vi "test purge with argon.vi"() -> ()   [LabVIEW 2017]
uses:
  <instrlib>/Harvard Apparatus PHD Ultra Series/Harvard Apparatus PHD Ultra Series.lvlib
panel:
  in  "VISA resource name":refnum<visa-resource-name>="COM12"
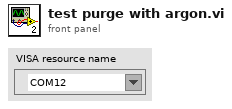
[diagram p1: front panel]
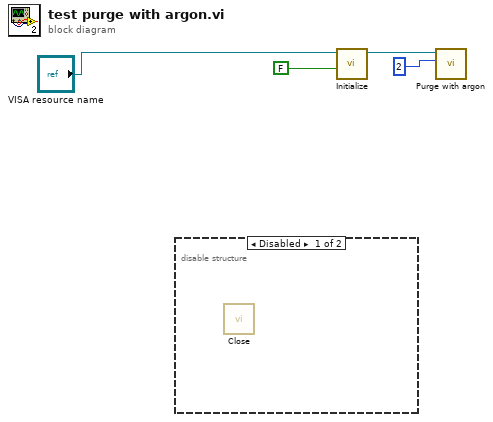
[diagram p0: block diagram]
diagram:
  n1 = disable-structure shown="Disabled" {
    frame Disabled {
      n2 = call <instrlib>:"Close.vi"() -> ()  [unwired: 11 in, 1 out]
    }
    frame Enabled {
    }
  }
  n3 = call <instrlib>:"Initialize.vi"("ID Query (True)"=FALSE, "VISA resource name"="VISA resource name") -> ("VISA resource name out"=w2:refnum<visa-resource-name>)  [unwired: 8 in, 1 out]
  n4 = call "Purge with argon.vi"("Repeat times"=2, "Pump 1 COM"=w2) -> ()  [unwired: 10 in]
